vi "Wait time calc sub vi for testing log.vi"(8 "error in (no error)":errorcluster, 9 "Input matrix":T1, 10 "Elapsed time (min)":dbl, 11 "Input column":i32) -> (0 "error out":errorcluster, 2 "Column out":i32, 3 "Wait time (min)":u32)   [LabVIEW 2010]
uses:
  <vilib>/Analysis/Matrix/Datatypes/RealMatrix.ctl
  <vilib>/Analysis/Matrix/NI_Matrix.lvlib
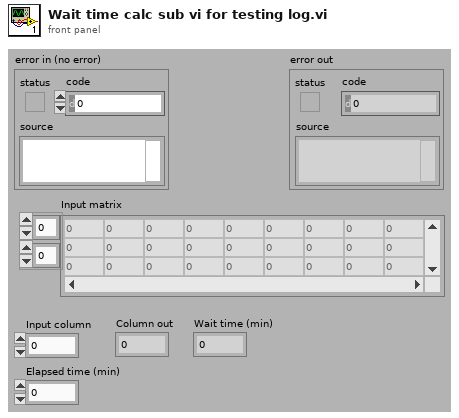
[diagram p1: front panel]
types:
  T1 = typedef "NI_Matrix.lvlib/RealMatrix.ctl" = dbl[][]
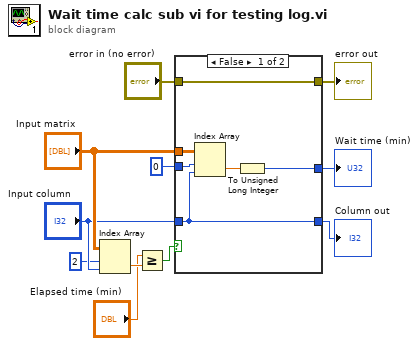
[diagram p0: block diagram]
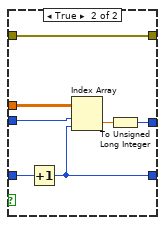
[diagram p2: hidden frame]
diagram:
  n1 = Index Array(array="Input matrix", index (row)=2, index (col)="Input column") -> (element=w11:dbl)
  n2 = Greater Or Equal?(x="Elapsed time (min)", y=w11) -> (x >= y?=w5:bool)
  n3 = case shown="False" w5 {
    tunnel: 0 -> [w17 w23]
    tunnel: "Input matrix" -> [w16 w24]
    tunnel: "Input column" -> [w13 w22]
    tunnel: [w14 w20] -> w8
    tunnel: [w13 w21] -> w7
    tunnel: [w12 w18] -> w1
    tunnel: "error in (no error)" -> [w12 w18]
    frame False {
      n4 = Index Array(array=w16, index (row)=w17, index (col)=w13) -> (element=w15:dbl)
      n5 = To Unsigned Long Integer(number=w15) -> (unsigned 32bit integer=w14:u32)
    }
    frame True {
      n6 = Increment(x=w22) -> (x+1=w21:i32)
      n7 = Index Array(array=w24, index (row)=w23, index (col)=w21) -> (element=w19:dbl)
      n8 = To Unsigned Long Integer(number=w19) -> (unsigned 32bit integer=w20:u32)
    }
  }
  "Column out" <- w7
  "Wait time (min)" <- w8
  "error out" <- w1
